vi "G_EQUIP_CMM.vi"() -> ()   [LabVIEW 2018]
panel:
  in  "semaphore":T1 caption="세마포어"
  out "G_EQUIP_CMM":T2
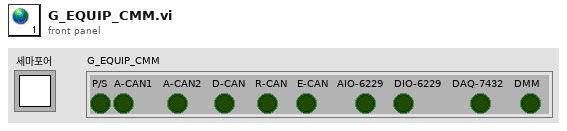
[diagram p1: front panel]
types:
  T1 = typedef "Semaphore RefNum" = refnum<k1>
  T2 = cluster{"P/S":bool, "A-CAN1":bool, "A-CAN2":bool, "D-CAN":bool, "R-CAN":bool, "E-CAN":bool, "AIO-6229":bool, "DIO-6229":bool, "DAQ-7432":bool, "DMM":bool}
diagram:
